vi "onProcessKilled.vi"(11 "SMO.Example in":refnum<class "SMO.Example.lvclass">) -> ()   [LabVIEW 2013, in "SMO.Example.lvclass"]
uses:
  SMO.Example.lvclass
  src/SMO/SMO.lvclass
panel:
  # "This method is called if the call chain of the SMO\nis leaving memory while the process is running.\nAssume all references created in non-critical reference\noverrides are invalid."
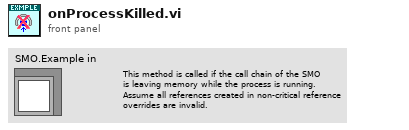
[diagram p1: front panel]
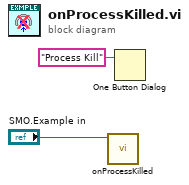
[diagram p0: block diagram]
diagram:
  n1 = call-parent "onProcessKilled.vi"("SMO in"="SMO.Example in") -> ()  [unwired: 11 in]
  n2 = One Button Dialog(message="Process Kill") -> ()  [unwired: 1 in, 1 out]
